vi "Set Calibration Coefficients.vi"(8 "Zero Value":dbl, 9 "Excitation Voltage":dbl, 10 "Calibration Factor":dbl, 11 "Channel Settings":T1) -> (3 "Updated Channel Settings":T1)   [LabVIEW 2021, in "Acquisition.lvlib"]
doc: "Set new calibration coefficients on 'Channel Settings'."
uses:
  Acquisition.lvlib
  Channel Settings.ctl
  IO Device.ctl
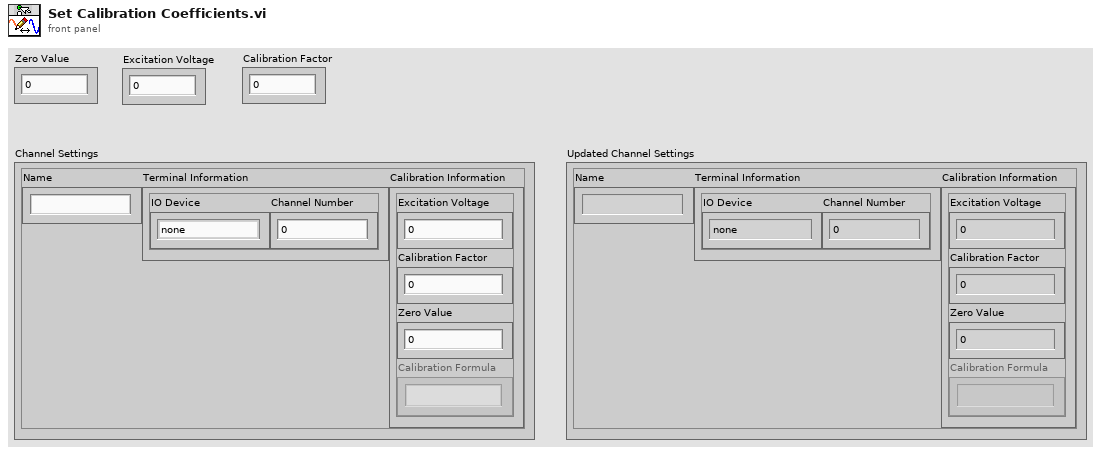
[diagram p1: front panel]
types:
  T1 = typedef "Acquisition.lvlib/Channel Settings.ctl" = cluster{"Name":string, "Terminal Information":cluster{"IO Device":T2, "Channel Number":i32}, "Calibration Information":cluster{"Excitation Voltage":dbl, "Calibration Factor":dbl, "Zero Value":dbl, "Calibration Formula":string}}
  T2 = typedef "Acquisition.lvlib/IO Device.ctl" = enum16{"none", "9219", "9401"}
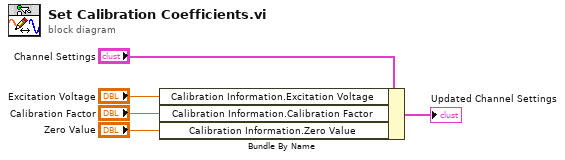
[diagram p0: block diagram]
diagram:
  n1 = Bundle By Name(cluster="Channel Settings", "Calibration Information.Excitation Voltage"="Excitation Voltage", "Calibration Information.Calibration Factor"="Calibration Factor", "Calibration Information.Zero Value"="Zero Value") -> (→"Updated Channel Settings":T1)
